vi "Query Minimum Sample Timer.vi"(8 "error in (no error)":errorcluster, 11 "VISA resource name":refnum<visa-resource-name>) -> (0 "error out":errorcluster, 2 "Minimum Sample Timer":dbl, 3 "VISA resource name out":refnum<visa-resource-name>)   [LabVIEW 2013, in "Agilent 3446X Series.lvlib"]
doc: "Query the \"MIN\" time for the sample timer.\n\n<b>Notes:</b>\n1) The value of MIN for the sample timer is measurement dependent. It depends on such things as the integration time, autozero on or off, autorange on or off, and the measurement range. Basically, MIN is automatically determined so that the sample interval is always greater than the sampling time.\n\n2) Execute this VI to determine the recommended interval for the current measurement configuration.\nSince the minimum value changes depending on configuration, a command order dependency exists.\nYou must completely configure the measurement before setting the sample timer to MIN, or you may\ngenerate an error. A complete configuration includes such things as math statistics or scaling.\n\n3) When using autorange, the MIN value is the recommended value, not the absolute minimum value.\nWith autorange enabled, MIN is calculated assuming a single range change will occur for every measurement (not multiple ranges, just one range up or down per measurement). You can specify an <interval> between the absolute minimum (assumes no range changes) and the recommended MIN value, but it may generate a timing violation error when making measurements. Applying a value less than the absolute minimum will generate an error.\nTo determine the absolute minimum value for the present configuration, set the sample time to 20 micro seconds (which may generate a settings conflict error), then read back the current sample timer value using the SAMPle:TIMer? query. The sample source must be set to timer with a sample count or trigger count greater than 1, for the settings conflict error to occur. The settings conflict error causes the timer to be set to the absolute minimum value.\n\n4) The sample time resolution is 1 micro seconds, the aperture resolution is 2 micro seconds, and the actual hardware resolution is not exactly 1 us. There are cases where a sample time value, rounded to the nearest hardware resolution, will result in a smaller value than aperture when rounded to 2 micro seconds. This will create error - 221,\"Settings conflict; cannot meet requested timing; SAMP:TIM changed\". For example, the following sequence of commands generates error -221 and sets the sample time to +2.00100000E-003."
uses:
  <instrlib>/Agilent 3446X Series/Agilent 3446X Series.lvlib
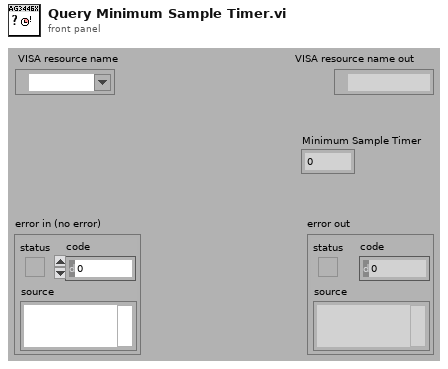
[diagram p1: front panel]
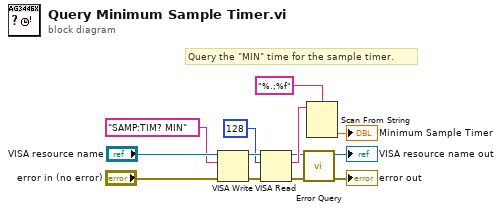
[diagram p0: block diagram]
diagram:
  # "Query the \"MIN\" time for the sample timer."
  n1 = VISA Write(VISA resource name="VISA resource name", write buffer="SAMP:TIM? MIN", error in (no error)="error in (no error)") -> (VISA resource name out=w7:refnum<visa-resource-name>, error out=w8:errorcluster)  [unwired: 1 out]
  n2 = VISA Read(VISA resource name=w7, byte count=u32 128, error in (no error)=w8) -> (VISA resource name out=w3:refnum<visa-resource-name>, read buffer=w6:string, error out=w2:errorcluster)  [unwired: 1 out]
  n3 = call <instrlib>:"Error Query.vi"("error in (no error)"=w2, "VISA resource name"=w3) -> ("error out"=→"error out":errorcluster, "VISA resource name out"=→"VISA resource name out":refnum<visa-resource-name>)  [unwired: 6 in, 2 out]
  n4 = Scan From String(format string="%.;%f", input string=w6) -> (output 1=→"Minimum Sample Timer":dbl)  [unwired: 3 in, 3 out]
